vi "Example2.vi"() -> ()   [LabVIEW 2023]
doc: "Simple example of file operations with write/read delimited spreadsheet."
uses:
  <vilib>/Utility/file.llb/Write Delimited Spreadsheet (DBL).vi
  <vilib>/Utility/file.llb/Read Delimited Spreadsheet (DBL).vi
panel:
  in  "Load":bool
  in  "Clear":bool
  out "Graph":dbl[](graph) caption="Obecny pomiar"
  in  "GetData":bool
  in  "SaveData":bool
  in  "stop":bool
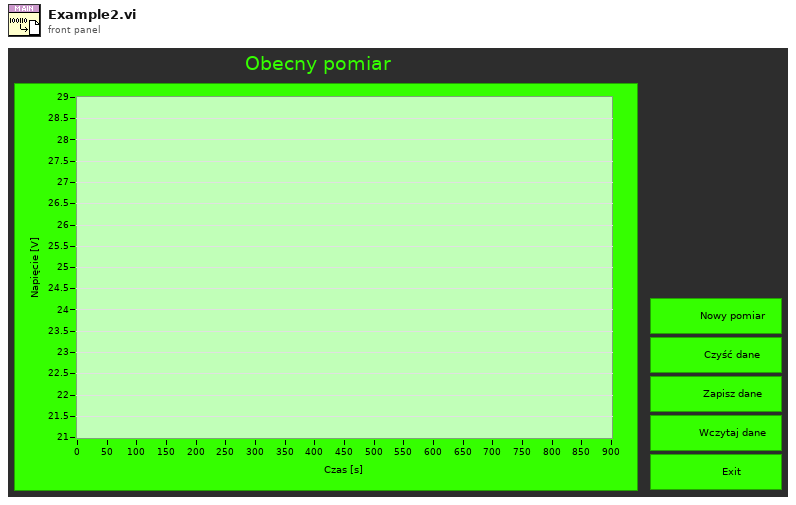
[diagram p1: front panel]
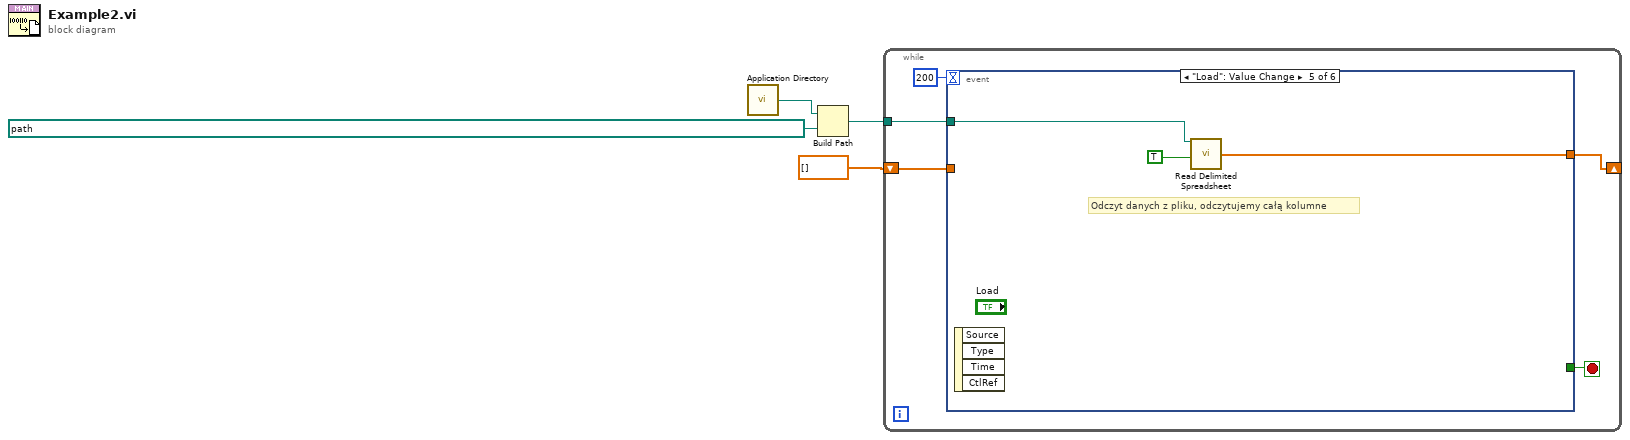
[diagram p0: block diagram]
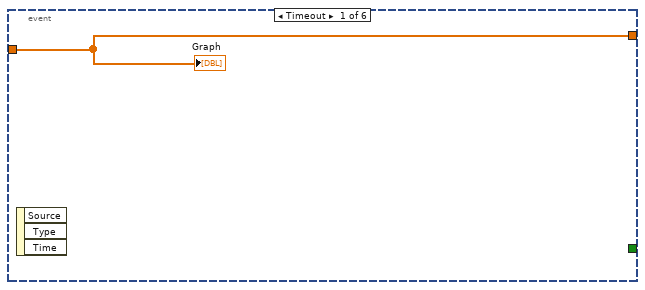
[diagram p2: hidden frame]
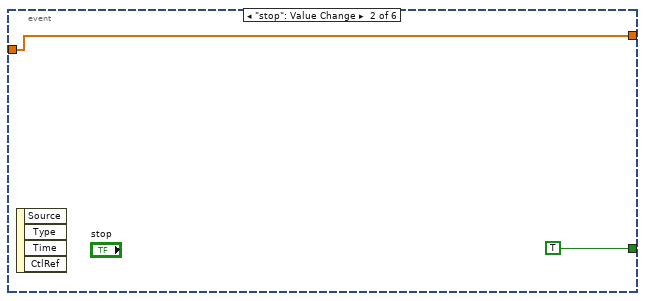
[diagram p3: hidden frame]
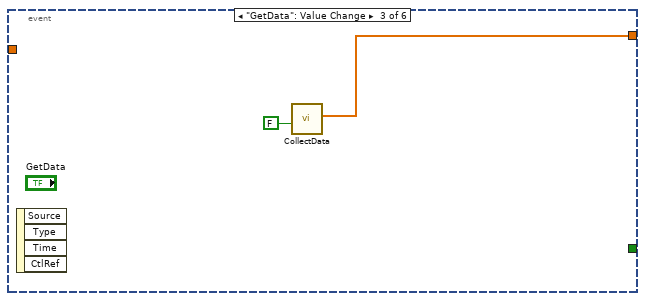
[diagram p4: hidden frame]
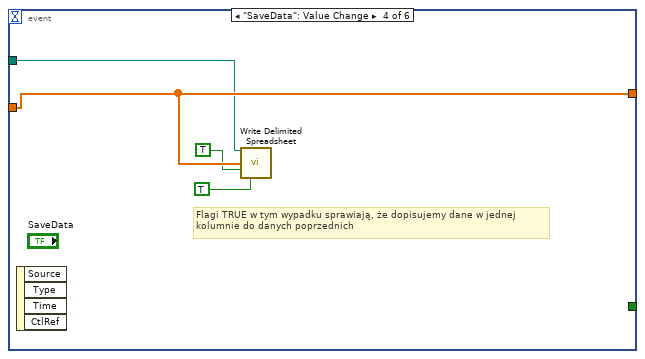
[diagram p5: hidden frame]
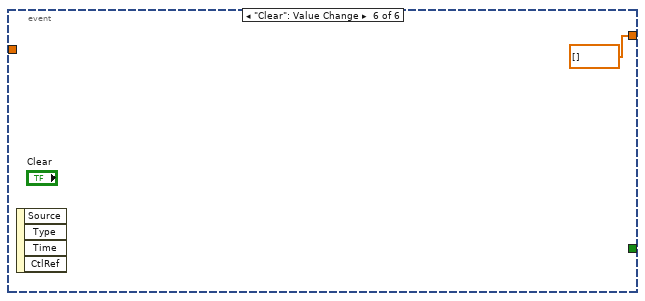
[diagram p6: hidden frame]
diagram:
  n1 = call <vilib>:"Application Directory.vi"() -> ("Application Directory"=w2:path)
  n2 = Build Path(base path=w2, name or relative path=path "C:/Users/Szymon Chmielewski/Desktop/NAUKA/STUDIA/SEMESTR 6/PwŚG/GSR_registers_and_RResp_labels/GSR_registers_and_RResp_labels/A1P.txt") -> (appended path=w1:path)
  n3 = while {
    shift-right: [w7] -> _
    shift-left: dbl[] [] -> [w8]
    tunnel: w1 -> [w6]
    stop <- w5 stop-if-true
    n4 = event shown="[4] \"Load\": Value Change" {
      selector: _ -> [_ _ _ _ _ _]
      dyn-events: _ -> [_ _ _ _ _ _]
      timeout: 200 -> [_ _ _ _ _ _]
      tunnel: w8 -> [w10 w11 _ w18 _ _]
      tunnel: [w10 w11 w14 w18 w21 dbl[] [] ("Data")] -> w7
      tunnel: [_ TRUE ("stop") _ _ _ _] -> w5
      tunnel: w6 -> [_ _ _ w15 w20 _]
      event Timeout {
        n5 = event-data() -> ()  [unwired: 1 in, 3 out]
        "Graph" <- w10
      }
      event "stop": Value Change {
        n6 = event-data() -> ()  [unwired: 1 in, 4 out]
      }
      event "GetData": Value Change {
        n7 = event-data() -> ()  [unwired: 1 in, 4 out]
        n8 = call "CollectData.vi"("SimErr"=FALSE) -> ("Data"=w14:dbl[])  [unwired: 5 in, 1 out]
      }
      event "SaveData": Value Change {
        # "Flagi TRUE w tym wypadku sprawiają, że dopisujemy dane w jednej\nkolumnie do danych poprzednich"
        n9 = event-data() -> ()  [unwired: 1 in, 4 out]
        n10 = call-poly <vilib>:"Write Delimited Spreadsheet.vi"("file path (dialog if empty)"=w15, "1D data"=w18, "append to file? (new file:F)"=TRUE, "transpose? (no:F)"=TRUE) -> ()  [unwired: 10 in, 2 out]
      }
      event "Load": Value Change {
        # "Odczyt danych z pliku, odczytujemy całą kolumne"
        n11 = event-data() -> ()  [unwired: 1 in, 4 out]
        n12 = call-poly <vilib>:"Read Delimited Spreadsheet.vi"("file path (dialog if empty)"=w20, "transpose? (F)"=TRUE) -> ("first row"=w21:dbl[])  [unwired: 8 in, 5 out]
      }
      event "Clear": Value Change {
        n13 = event-data() -> ()  [unwired: 1 in, 4 out]
      }
    }
  }
